vi "Set Robot Position.vi"(10 "setpoint y":dbl format="%.2f", 11 "setpoint x":dbl format="%.2f") -> ()   [LabVIEW 2015]
uses:
  Vision/Vision Global.vi
  <vilib>/addons/control/pid/pid.llb/PID (DBL).vi
  <vilib>/addons/control/pid/NI_PID_pid.lvlib
panel:
  in  "PID x":T1={"proportional gain (Kc)"=1.0, "integral time (Ti, min)"=0.01, "derivative time (Td, min)"=0.0} {"derivative time (Td, min)" format="%.3f"; "integral time (Ti, min)" format="%.3f"; "proportional gain (Kc)" format="%.3f"}
  in  "PID y":T1={"proportional gain (Kc)"=1.0, "integral time (Ti, min)"=0.01, "derivative time (Td, min)"=0.0} {"derivative time (Td, min)" format="%.3f"; "integral time (Ti, min)" format="%.3f"; "proportional gain (Kc)" format="%.3f"}
  out "Numeric":dbl
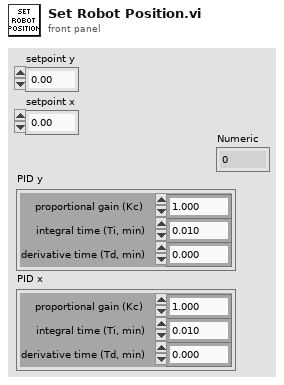
[diagram p1: front panel]
types:
  T1 = cluster{"proportional gain (Kc)":dbl, "integral time (Ti, min)":dbl, "derivative time (Td, min)":dbl}
  T2 = cluster{"Distance (ft)":dbl, "Center":cluster{dbl, dbl}, "Normalized Rect":cluster{"Numeric":dbl, "Numeric 2":dbl, "Numeric 3":dbl, "Numeric 5":dbl}}[]
  T3 = cluster{"Distance (ft)":dbl, "Center":cluster{dbl, dbl}, "Normalized Rect":cluster{"Numeric":dbl, "Numeric 2":dbl, "Numeric 3":dbl, "Numeric 5":dbl}}
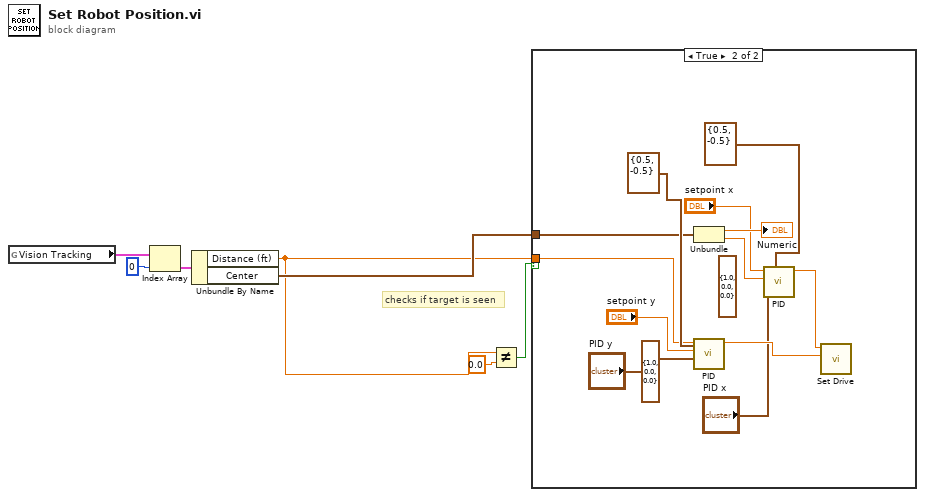
[diagram p0: block diagram]
diagram:
  # "checks if target is seen"
  n1 = global read "Vision Global.vi" "Vision Tracking"() -> (w5:T2)
  n2 = Index Array(array=w5, index=0) -> (element=w6:T3)
  n3 = Unbundle By Name(w6) -> ("Distance (ft)"=w2:dbl, "Center"=w4:cluster{dbl, dbl})
  n4 = Not Equal?(x=w2, y=0.0) -> (x != y?=w1:bool)
  n5 = case shown="True" w1 {
    tunnel: w4 -> [_ w17]
    tunnel: w2 -> [_ w8]
    frame False {
    }
    frame True {
      (unwired) T1 {"proportional gain (Kc)"=1.0, "integral time (Ti, min)"=0.0, "derivative time (Td, min)"=0.0} ("PID gains")
      (unwired) T1 {"proportional gain (Kc)"=1.0, "integral time (Ti, min)"=0.0, "derivative time (Td, min)"=0.0} ("PID gains")
      n6 = Unbundle(w17) -> (→"Numeric":dbl, w16:dbl)
      n7 = call-poly <vilib>:"PID.vi"("output range"=cluster{"output high":dbl, "output low":dbl} {"output high"=0.5, "output low"=-0.5}, "PID gains"="PID y", "process variable"="setpoint y", "setpoint"=w8) -> ("output"=w13:dbl)  [unwired: 6 in, 1 out]
      n8 = call-poly <vilib>:"PID.vi"("output range"=cluster{"output high":dbl, "output low":dbl} {"output high"=0.5, "output low"=-0.5}, "PID gains"="PID x", "process variable"=w16, "setpoint"="setpoint x") -> ("output"=w14:dbl)  [unwired: 6 in, 1 out]
      n9 = call "Set Drive.vi"("Y axis value"=w13, "X axis value"=w14) -> ()  [unwired: 10 in]
    }
  }
